vi "Create Message - Periodic And Trigger_ex.vi"() -> ()   [LabVIEW 2019]
uses:
  <vilib>/NI VeriStand/Custom Device API/Custom Device Item Ref.ctl
  Control 3.ctl
  Control 4.ctl
  Scripting API/Polymorphic/Create Message_PeriodicAndTrigger.vi
  Scripting API/Scripting API.lvlib
  <vilib>/NI VeriStand/Custom Device API/Custom Device API.lvlib
panel:
  out "Message Group Refnum Out":T1=18446744073709551615 format="%.0x"
  out "Message Refnum":T1=18446744073709551615 format="%.0x"
  out "Error Out":errorcluster
  in  "Message Group Refnum In":T1=18446744073709551615 format="%.0x"
  in  "Message Name":string
  in  "Period (sec)":u32
  in  "Error In":errorcluster
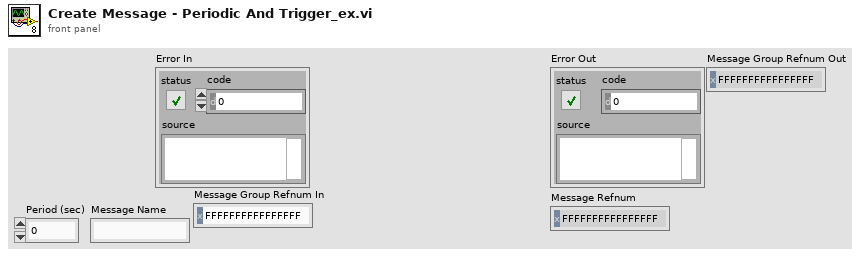
[diagram p1: front panel]
types:
  T1 = typedef "Custom Device API.lvlib/Custom Device Item Ref.ctl" = u64
  T2 = typedef "Control 3.ctl" = cluster{"Protection":T3, "Enable Periodic Default":bool, "Trigger Channel Refnum":T1}
  T3 = typedef "Control 4.ctl" = enum16{"None", "CRC-32", "Checksum U8", "Checksum U16", "Checksum U32"}
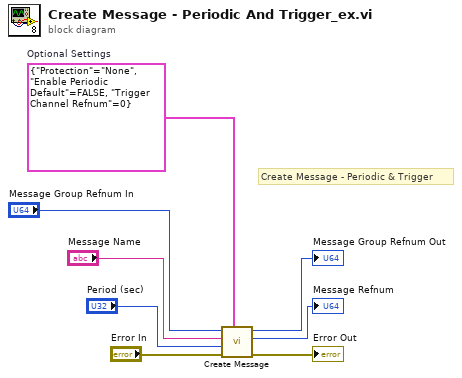
[diagram p0: block diagram]
diagram:
  w1 = T2 {"Protection"=enum."None", "Enable Periodic Default"=FALSE, "Trigger Channel Refnum"=0}  # Optional Settings
  # "Create Message - Periodic & Trigger"
  n1 = call-poly "Create Message.vi"("Optional Settings"=w1, "Error In"="Error In", "Period (sec)"="Period (sec)", "Message Name"="Message Name", "Message Group Refnum In"="Message Group Refnum In") -> ("Error Out"=→"Error Out":errorcluster, "Message Refnum"=→"Message Refnum":T1, "Message Group Refnum Out"=→"Message Group Refnum Out":T1)  [unwired: 4 in]
